vi "User Events - DeInit.vi"(8 "error in (no error)":errorcluster, 11 "UE Data Container":T1) -> (0 "error out":errorcluster)   [LabVIEW 2017]
doc: "De - Initialize all user events for ATM Controller."
uses:
  UE Data Container.ctl
  Error Handler/Controls/Error Data.ctl
  UIs/User Console/Controls/User Console - Transaction Enum.ctl
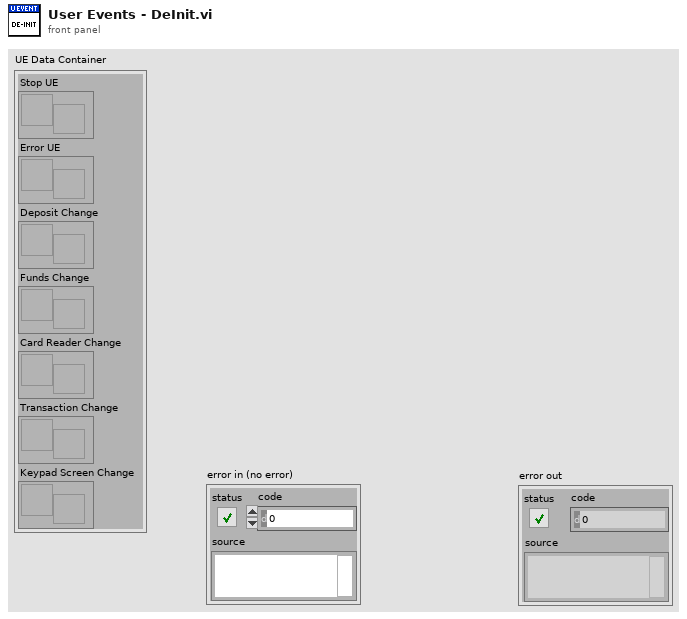
[diagram p1: front panel]
types:
  T1 = typedef "UE Data Container.ctl" = cluster{"Stop UE":refnum<user-event>, "Error UE":refnum<user-event>, "Deposit Change":refnum<user-event>, "Funds Change":refnum<user-event>, "Card Reader Change":refnum<user-event>, "Transaction Change":refnum<user-event>, "Keypad Screen Change":refnum<user-event>}
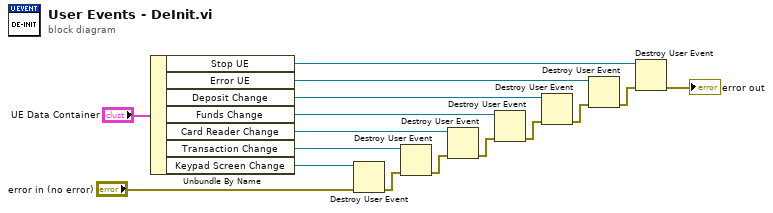
[diagram p0: block diagram]
diagram:
  n1 = Unbundle By Name("UE Data Container") -> ("Stop UE"=w9:refnum<user-event>, "Error UE"=w10:refnum<user-event>, "Deposit Change"=w11:refnum<user-event>, "Funds Change"=w12:refnum<user-event>, "Card Reader Change"=w13:refnum<user-event>, "Transaction Change"=w14:refnum<user-event>, "Keypad Screen Change"=w15:refnum<user-event>)
  n2 = Destroy User Event(user event=w15, error in="error in (no error)") -> (error out=w7:errorcluster)
  n3 = Destroy User Event(user event=w14, error in=w7) -> (error out=w6:errorcluster)
  n4 = Destroy User Event(user event=w13, error in=w6) -> (error out=w5:errorcluster)
  n5 = Destroy User Event(user event=w12, error in=w5) -> (error out=w4:errorcluster)
  n6 = Destroy User Event(user event=w11, error in=w4) -> (error out=w3:errorcluster)
  n7 = Destroy User Event(user event=w10, error in=w3) -> (error out=w2:errorcluster)
  n8 = Destroy User Event(user event=w9, error in=w2) -> (error out=→"error out":errorcluster)
